vi "S2C_5190CR_Proc_SendCmd.vi"(8 "Error In":errorcluster, 9 "ExeRef":refnum<vi>, 11 "Q-Ref":refnum<queue>) -> (0 "Error Out":errorcluster, 3 "Command":string)   [LabVIEW 2015]
doc: "Custom VI designed to request the Current, Power, or Voltage for a specific outlet."
uses:
  S2C_5190CR_Proc_Globals.vi
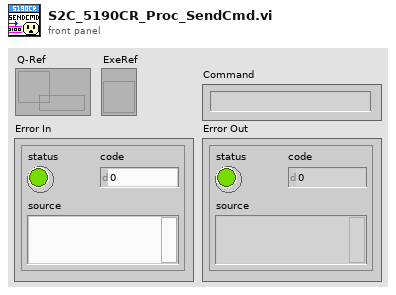
[diagram p1: front panel]
types:
  T1 = cluster{"Caller-Q":refnum<queue>, "Command":string, "Return":string, "Data":variant, "Timeout":dbl}
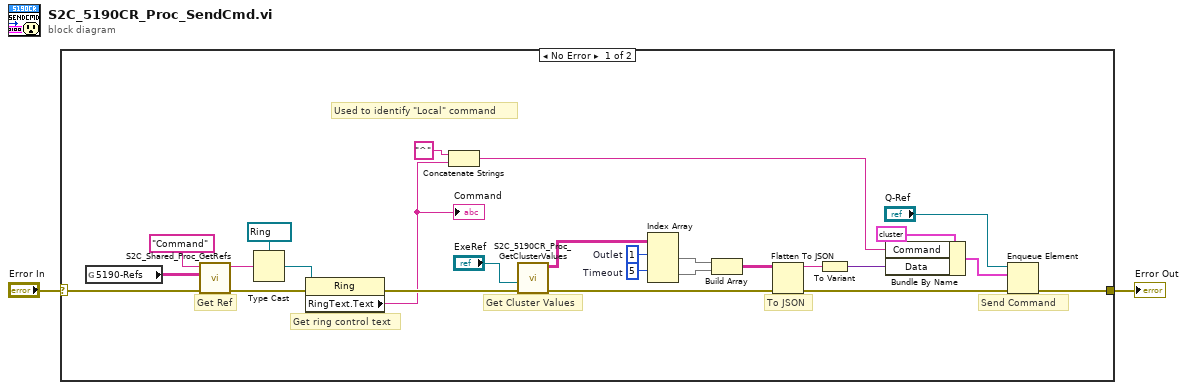
[diagram p0: block diagram]
diagram:
  n1 = case shown="No Error" "Error In" {
    selector: "Error In" -> [w18 w29]
    tunnel: [w26 w29] -> w1
    frame No Error {
      w4 = 5  # Timeout
      w5 = 1  # Outlet
      # "Get Cluster Values"
      # "To JSON"
      # "Get ring control text"
      # "Get Ref"
      # "Used to identify \"Local\" command"
      # "Send Command"
      n2 = global read "S2C_5190CR_Proc_Globals.vi" "5190-Refs"() -> (w16:string[][])
      n3 = call "S2C_Shared_Proc_GetRefs.vi"("Error In"=w18, "Refs"=w16, "Label"="Command") -> ("Error Out"=w19:errorcluster, "Reference"=w22:string)  [unwired: 7 in]
      n4 = Type Cast(type=refnum<vi> refnum ("Enum"), x=w22) -> (*(type *) &x=w20:refnum<vi>)
      n5 = property class="Ring"(reference=w20, error in=w19) -> (error out=w12:errorcluster, "RingText.Text"=w3:string)  [unwired: 1 out]
      "Command" <- w3
      n6 = Concatenate Strings("^" ("string"), w3) -> (w23:string)
      n7 = call "S2C_5190CR_Proc_GetClusterValues.vi"("Error In"=w12, "ExeRef"="ExeRef") -> ("Error Out"=w11:errorcluster, "Settings"=w10:string[][])  [unwired: 8 in]
      n8 = Index Array(array=w10, index (row) #1=w5, index (row) #2=w4) -> (element #1=w8:string[], element #2=w9:string[])  [unwired: 2 in]
      n9 = Build Array(w8, w9) -> (w7:string[][])
      n10 = Flatten To JSON(anything=w7, error in (no error)=w11) -> (JSON string=w15:string, 11:w13:errorcluster)  [unwired: 1 in]
      n11 = To Variant(anything=w15) -> (Variant=w14:variant)
      n12 = Bundle By Name(cluster=T1 {"Caller-Q"=refnum, "Command"="", "Return"="Local", "Data"=variant, "Timeout"=10.0} ("element"), "Command"=w23, "Data"=w14) -> (w25:T1)
      n13 = Enqueue Element(queue="Q-Ref", element=w25, error in (no error)=w13) -> (error out=w26:errorcluster)  [unwired: 1 in, 2 out]
    }
    frame Error {
    }
  }
  "Error Out" <- w1
